vi "Measurement Logic.vi"() -> ()   [LabVIEW 2020, in "NIDigitalBurstPattern.lvlib"]
uses:
  NIDigitalBurstPattern.lvlib
  Measurement Configuration.ctl
  Measurement Results.ctl
  <instrlib>/niDigital/niDigital.llb/niDigital History RAM Cycle Information (1D Pin States).ctl
  <instrlib>/niDigital/niDigital.llb/niDigital Pin State.ctl
  <vilib>/MeasurementLink/MeasurementLink Measurement Server/Classes/MeasurementContext/MeasurementContext.lvclass
  Measurement Service Helpers/Reserve (1 Session).vi
  Measurement Service Helpers/Unreserve (1 Session).vi
  Measurement Service Helpers/Measurement Service Helpers.lvlib
panel:
  out "Measurement Context out":refnum<class "MeasurementContext.lvclass">
  in  "Measurement Context":refnum<class "MeasurementContext.lvclass">
  out "Measurement Results":T1 {"HRAM information"."actual pin states" items=["0"=0, "1"=1, "L"=3, "H"=4, "X"=5, "M"=6, "V"=7, "D"=8, "E"=9, "Not A Pin State"=254, "Pin State Not Acquired"=255]; "HRAM information"."expected pin states" items=["0"=0, "1"=1, "L"=3, "H"=4, "X"=5, "M"=6, "V"=7, "D"=8, "E"=9, "Not A Pin State"=254, "Pin State Not Acquired"=255]}
  in  "Measurement Configuration":T4
  out "error out":errorcluster
  in  "error in":errorcluster
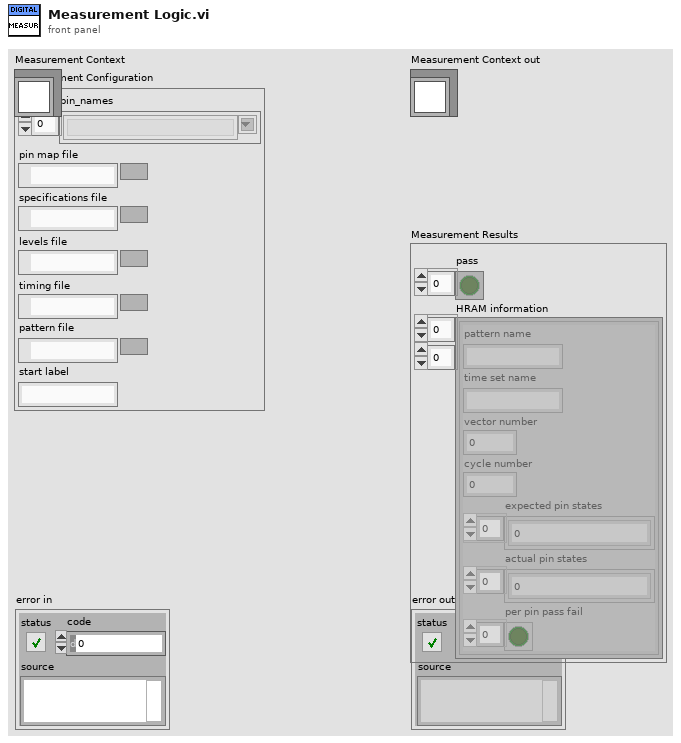
[diagram p1: front panel]
types:
  T1 = typedef "NIDigitalBurstPattern.lvlib/Measurement Results.ctl" = cluster{"pass":bool[], "HRAM information":T2[][]}
  T2 = typedef "niDigital History RAM Cycle Information (1D Pin States).ctl" = cluster{"pattern name":string, "time set name":string, "vector number":i64, "cycle number":i64, "expected pin states":T3[], "actual pin states":T3[], "per pin pass fail":bool[]}
  T3 = typedef "niDigital Pin State.ctl" = u8
  T4 = typedef "NIDigitalBurstPattern.lvlib/Measurement Configuration.ctl" = cluster{"pin_names":string[], "pin map file":path, "specifications file":path, "levels file":path, "timing file":path, "pattern file":path, "start label":string}
  T5 = typedef "Measurement Service Helpers.lvlib/GRPC Clients.ctl" = cluster{"discovery service gRPC ID":T6, "session manager service gRPC ID":T6}
  T6 = typedef "grpc-lvsupport-release.lvlib/grpcId.ctl" = u64
  T7 = typedef "MeasurementLink Session Management Client.lvlib/ni_measurementlink_sessionmanagement_v1_SessionInformation.ctl" = cluster{"session":T8, "resource_name":string, "channel_list":string, "instrument_type_id":string, "session_exists":bool, "channel_mappings":T9[]}
  T8 = typedef "MeasurementLink Session Management Client.lvlib/nidevice_grpc_Session.ctl" = cluster{"name":string}
  T9 = typedef "MeasurementLink Session Management Client.lvlib/ni_measurementlink_sessionmanagement_v1_ChannelMapping.ctl" = cluster{"pin_or_relay_name":string, "site":i32, "channel":string}
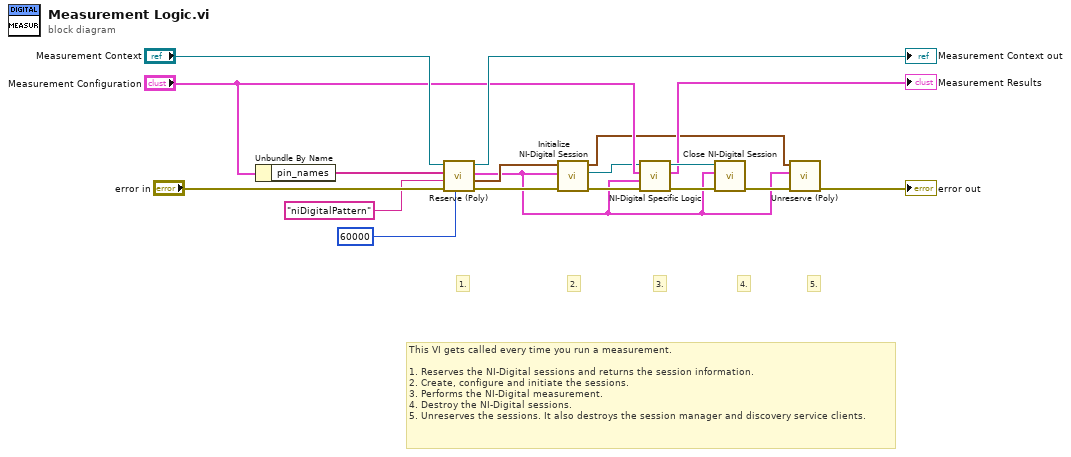
[diagram p0: block diagram]
diagram:
  # "This VI gets called every time you run a measurement.\n\n1. Reserves the NI-Digital sessions and returns the session information.\n2. Create, configure and initiate the sessions.\n3. Performs the NI-Digital measurement.\n4. Destroy the NI-Digital sessions.\n5. Unreserves the sessions. It also destroys the session manager and discovery service clients."
  # "5."
  # "4."
  # "3."
  # "2."
  # "1."
  n1 = Unbundle By Name("Measurement Configuration") -> ("pin_names"=w15:string[])
  n2 = call-poly "Reserve (Poly).vi"("timeout in milliseconds"=60000, "error in"="error in", "instrument type ID"="niDigitalPattern", "pin or relay names"=w15, "Measurement Context In"="Measurement Context") -> ("error out"=w16:errorcluster, "gRPC clients out"=w3:T5, "session information"=w2:T7, "Measurement Context out"=→"Measurement Context out":refnum<class "MeasurementContext.lvclass">)  [unwired: 3 in]
  n3 = call "Initialize NI-Digital Session.vi"("error in (no error)"=w16, "session information"=w2, "gRPC clients"=w3) -> ("error out"=w12:errorcluster, "instrument handle"=w1:refnum<k15>, "gRPC clients out"=w4:T5)  [unwired: 6 in]
  n4 = call "NI-Digital Specific Logic.vi"("error in"=w12, "session information"=w2, "Measurement Configuration"="Measurement Configuration", "instrument handle"=w1) -> ("error out"=w18:errorcluster, "Measurement Results"=→"Measurement Results":T1, "instrument handle out"=w7:refnum<k15>)  [unwired: 5 in]
  n5 = call "Close NI-Digital Session.vi"("error in (no error)"=w18, "session information"=w2, "instrument handle"=w7) -> ("error out"=w10:errorcluster)  [unwired: 8 in]
  n6 = call-poly "Unreserve (Poly).vi"("error in"=w10, "session information"=w2, "gRPC clients"=w4) -> ("error out"=→"error out":errorcluster)  [unwired: 8 in]
